vi "OE1022D_Query_Data.vi"(6 "错误输入（无错误）":errorcluster, 9 "VISA resource name":refnum<visa-resource-name>) -> (0 "error out":errorcluster, 1 "输出簇ADC":T2, 2 "输出簇B":T1, 3 "VISA resource name out":refnum<visa-resource-name>, 4 "输出簇A":T3)   [LabVIEW 2021]
doc: "Configures the reference source and the internal oscillator."
panel:
  out "AUX-ADC4 (V)":sgl format="%.3f"
  out "AUX-ADC3 (V)":sgl format="%.3f"
  out "AUX-ADC1 (V)":sgl format="%.3f"
  out "AUX-ADC2 (V)":sgl format="%.3f"
  out "R":sgl caption="R (Vrms)" format="%.3p"
  out "X":sgl caption="X (Vrms)" format="%.3p"
  out "Y":sgl caption="Y (Vrms)" format="%.3p"
  out "θ (°)":sgl caption="θ (deg)" format="%.2f"
  out "频率 (Hz)":sgl caption="Freq (Hz)" format="%#.3f"
  out "噪声":sgl caption="Noise(Vrms)" format="%.3p"
  out "Rh1":sgl caption="Rh1 (Vrms)" format="%.3p"
  out "θh1 (°)":sgl caption="θh1 (deg)" format="%.2f"
  out "Rh2":sgl caption="Rh2 (Vrms)" format="%.3p"
  out "Xh2":sgl caption="Xh2 (Vrms)" format="%.3p"
  out "Yh2":sgl caption="Yh2 (Vrms)" format="%.3p"
  out "θh2 (°)":sgl caption="θh2 (deg)" format="%.2f"
  out "Xh1":sgl caption="Xh1 (Vrms)" format="%.3p"
  out "Yh1":sgl caption="Yh1 (Vrms)" format="%.3p"
  out "X 2":sgl caption="X (Vrms)" format="%.3p"
  out "θh2 (°) 2":sgl caption="θh2 (deg)" format="%.2f"
  out "Y 2":sgl caption="Y (Vrms)" format="%.3p"
  out "R 2":sgl caption="R (Vrms)" format="%.3p"
  out "θ (°) 2":sgl caption="θ (deg)" format="%.2f"
  out "频率 (Hz) 2":sgl caption="Freq (Hz)" format="%#.3f"
  out "噪声 2":sgl caption="Noise(Vrms)" format="%.3p"
  out "Rh2 2":sgl caption="Rh2 (Vrms)" format="%.3p"
  out "Yh2 2":sgl caption="Yh2 (Vrms)" format="%.3p"
  out "Xh2 2":sgl caption="Xh2 (Vrms)" format="%.3p"
  out "Xh1 2":sgl caption="Xh1 (Vrms)" format="%.3p"
  out "Yh1 2":sgl caption="Yh1 (Vrms)" format="%.3p"
  out "Rh1 2":sgl caption="Rh1 (Vrms)" format="%.3p"
  out "θh1 (°) 2":sgl caption="θh1 (deg)" format="%.2f"
  in  "数据转换":u8[](array[numeric])
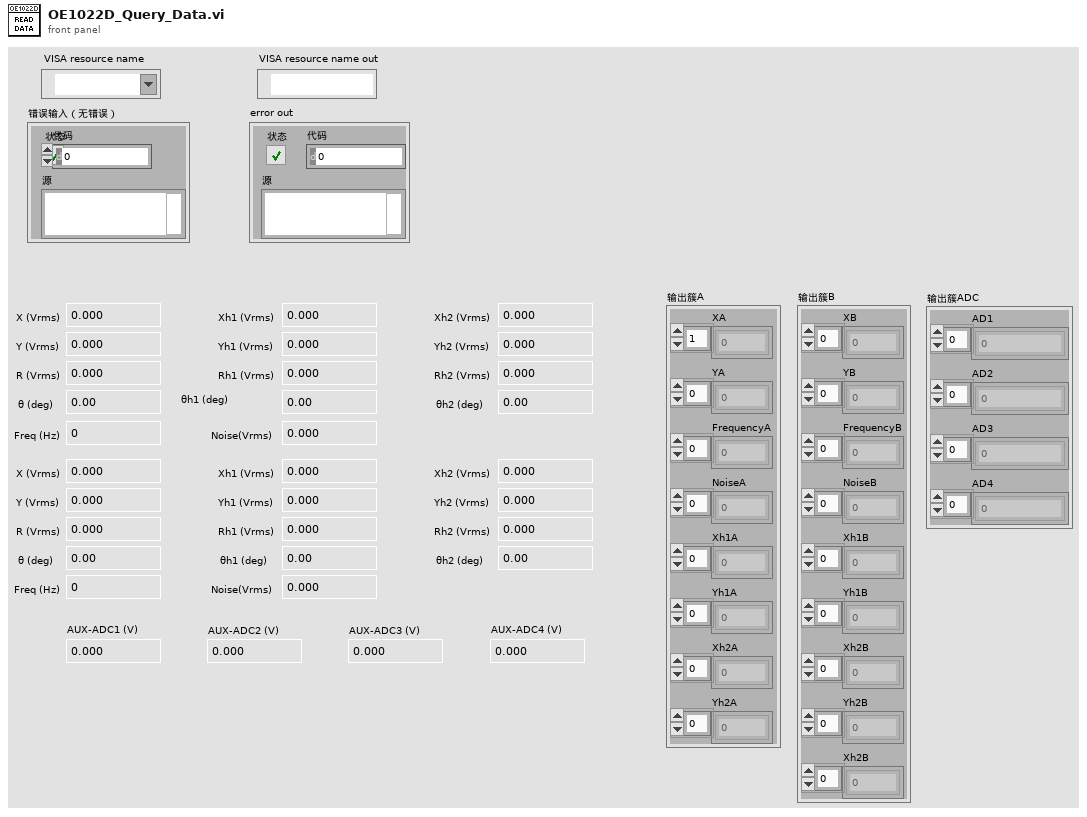
[diagram p1: front panel]
types:
  T1 = cluster{"XB":dbl[], "YB":dbl[], "FrequencyB":dbl[], "NoiseB":dbl[], "Xh1B":dbl[], "Yh1B":dbl[], "Xh2B":dbl[], "Yh2B":dbl[], "Xh2B":dbl[]}
  T2 = cluster{"AD1":dbl[], "AD2":dbl[], "AD3":dbl[], "AD4":dbl[]}
  T3 = cluster{"XA":dbl[], "YA":dbl[], "FrequencyA":dbl[], "NoiseA":dbl[], "Xh1A":dbl[], "Yh1A":dbl[], "Xh2A":dbl[], "Yh2A":dbl[]}
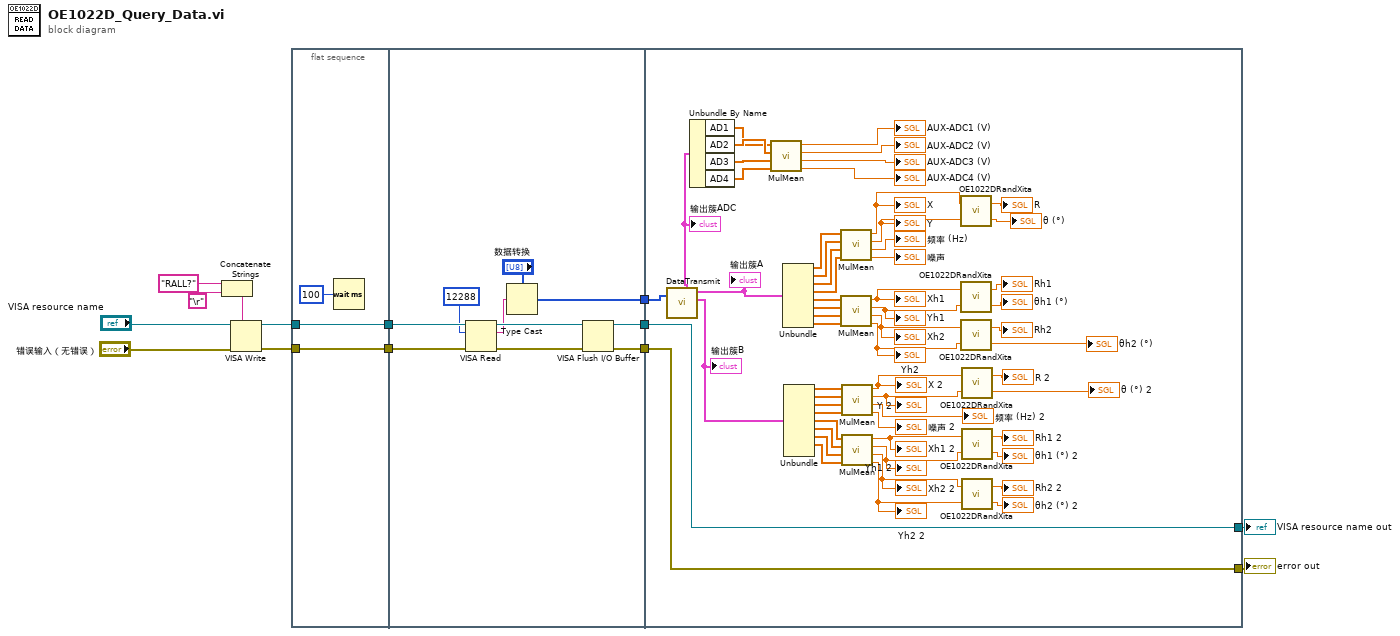
[diagram p0: block diagram]
diagram:
  n1 = Concatenate Strings("RALL?" ("命令输入"), "\r") -> (w13:string)
  n2 = VISA Write(VISA resource name="VISA resource name", write buffer=w13, error in (no error)="错误输入（无错误）") -> (VISA resource name out=w11:refnum<visa-resource-name>, error out=w9:errorcluster)  [unwired: 1 out]
  n3 = flat-sequence {
    tunnel: w11 -> [w16]
    tunnel: [w16] -> w10
    tunnel: w9 -> [w15]
    tunnel: [w15] -> w8
    tunnel: w10 -> [w25]
    tunnel: w8 -> [w24]
    tunnel: [w20] -> w7
    tunnel: [w19] -> w5
    tunnel: [w18] -> w3
    tunnel: w7 -> [w31]
    tunnel: [w30] -> w6
    tunnel: w5 -> [w30]
    tunnel: [w29] -> w4
    tunnel: w3 -> [w29]
    frame #0 {
      n4 = Wait (ms)(milliseconds to wait=u32 100 ("等待时间（毫秒）")) -> ()  [unwired: 1 out]
    }
    frame #1 {
      n5 = VISA Read(VISA resource name=w25, byte count=12288, error in (no error)=w24) -> (VISA resource name out=w27:refnum<visa-resource-name>, read buffer=w23:string, error out=w26:errorcluster)  [unwired: 1 out]
      n6 = Type Cast(type="数据转换", x=w23) -> (*(type *) &x=w20:u8[])
      n7 = VISA Flush I/O Buffer(VISA resource name=w27, error in (no error)=w26) -> (VISA resource name out=w19:refnum<visa-resource-name>, error out=w18:errorcluster)  [unwired: 1 in]
    }
    frame #2 {
      n8 = call <instrlib>:"DataTransmit.vi"("数据输入"=w31) -> ("输出簇ADC"=w81:T2, "输出簇A"=w28:T3, "输出簇B"=w66:T1)  [unwired: 2 in, 2 out]
      "输出簇A" <- w28
      "输出簇ADC" <- w81
      "输出簇B" <- w66
      n9 = Unbundle By Name(w81) -> ("AD1"=w82:dbl[], "AD2"=w83:dbl[], "AD3"=w84:dbl[], "AD4"=w85:dbl[])
      n10 = call <instrlib>:"MulMean.vi"("IN 4"=w85, "IN 3"=w84, "IN 2"=w83, "IN 1"=w82) -> ("mean 4"=→"AUX-ADC4 (V)":dbl, "mean 3"=→"AUX-ADC3 (V)":dbl, "mean 2"=→"AUX-ADC2 (V)":dbl, "mean 1"=→"AUX-ADC1 (V)":dbl)  [unwired: 4 in]
      n11 = Unbundle(w28) -> ("XA"=w36:dbl[], "YA"=w37:dbl[], "FrequencyA"=w38:dbl[], "NoiseA"=w39:dbl[], "Xh1A"=w46:dbl[], "Yh1A"=w47:dbl[], "Xh2A"=w48:dbl[], "Yh2A"=w49:dbl[])
      n12 = Unbundle(w66) -> ("XB"=w65:dbl[], "YB"=w64:dbl[], "FrequencyB"=w63:dbl[], "NoiseB"=w62:dbl[], "Xh1B"=w61:dbl[], "Yh1B"=w60:dbl[], "Xh2B"=w59:dbl[], "Yh2B"=w58:dbl[])  [unwired: 1 out]
      n13 = call <instrlib>:"MulMean.vi"("IN 4"=w39, "IN 3"=w38, "IN 2"=w37, "IN 1"=w36) -> ("mean 4"=→"噪声":dbl, "mean 3"=→"频率 (Hz)":dbl, "mean 2"=w42:dbl, "mean 1"=w41:dbl)  [unwired: 4 in]
      "X" <- w41
      "Y" <- w42
      n14 = call <instrlib>:"MulMean.vi"("IN 4"=w49, "IN 3"=w48, "IN 2"=w47, "IN 1"=w46) -> ("mean 4"=w55:dbl, "mean 3"=w54:dbl, "mean 2"=w51:dbl, "mean 1"=w50:dbl)  [unwired: 4 in]
      "Xh2" <- w54
      "Yh2" <- w55
      "Xh1" <- w50
      "Yh1" <- w51
      n15 = call <instrlib>:"MulMean.vi"("IN 4"=w62, "IN 3"=w63, "IN 2"=w64, "IN 1"=w65) -> ("mean 4"=→"噪声 2":dbl, "mean 3"=→"频率 (Hz) 2":dbl, "mean 2"=w72:dbl, "mean 1"=w71:dbl)  [unwired: 4 in]
      "X 2" <- w71
      "Y 2" <- w72
      n16 = call <instrlib>:"MulMean.vi"("IN 4"=w58, "IN 3"=w59, "IN 2"=w60, "IN 1"=w61) -> ("mean 4"=w78:dbl, "mean 3"=w77:dbl, "mean 2"=w74:dbl, "mean 1"=w73:dbl)  [unwired: 4 in]
      "Yh2 2" <- w78
      "Xh2 2" <- w77
      "Xh1 2" <- w73
      "Yh1 2" <- w74
      n17 = call <instrlib>:"OE1022DRandXita.vi"("Y"=w42, "X"=w41) -> ("θ (°)"=→"θ (°)":dbl, "R"=→"R":dbl)
      n18 = call <instrlib>:"OE1022DRandXita.vi"("Y"=w51, "X"=w50) -> ("θ (°)"=→"θh1 (°)":dbl, "R"=→"Rh1":dbl)
      n19 = call <instrlib>:"OE1022DRandXita.vi"("Y"=w55, "X"=w54) -> ("θ (°)"=→"θh2 (°)":dbl, "R"=→"Rh2":dbl)
      n20 = call <instrlib>:"OE1022DRandXita.vi"("Y"=w72, "X"=w71) -> ("θ (°)"=→"θ (°) 2":dbl, "R"=→"R 2":dbl)
      n21 = call <instrlib>:"OE1022DRandXita.vi"("Y"=w74, "X"=w73) -> ("θ (°)"=→"θh1 (°) 2":dbl, "R"=→"Rh1 2":dbl)
      n22 = call <instrlib>:"OE1022DRandXita.vi"("Y"=w78, "X"=w77) -> ("θ (°)"=→"θh2 (°) 2":dbl, "R"=→"Rh2 2":dbl)
    }
  }
  "VISA resource name out" <- w6
  "error out" <- w4
